vi "Script Classes in Acquire Method.vi"(8 "error in (no error)":errorcluster, 9 "Path":path, 10 "Project in":refnum<vi>, 11 "MeasurementMetaData in":refnum<class "MeasurementMetaData.lvclass">) -> (0 "error out":errorcluster, 3 "MeasurementMetaData out":refnum<class "MeasurementMetaData.lvclass">)   [LabVIEW 2016, in "MeasurementMetaData.lvclass"]
uses:
  MeasurementMetaData.lvclass
  MeasurementMetaData.lvclass/MeasurementMetaData.ctl
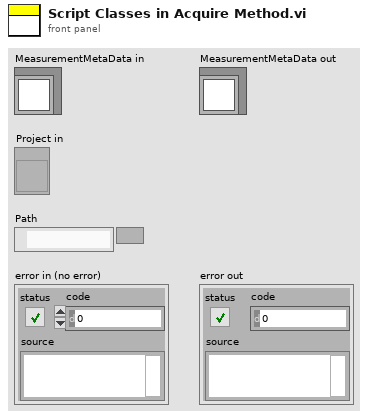
[diagram p1: front panel]
types:
  T1 = typedef "MeasurementMetaData.lvclass/Plugin Settings.ctl" = cluster{"Override Configure Method":bool, "Generate Custom Results Object":bool, "Override Measure Method":bool, "Override Close Method":bool, "Scope?":bool, "DMM?":bool, "FGEN?":bool, "PSU?":bool, "Acquisition Mode":enum16{"Continuous", "Single-Shot"}}
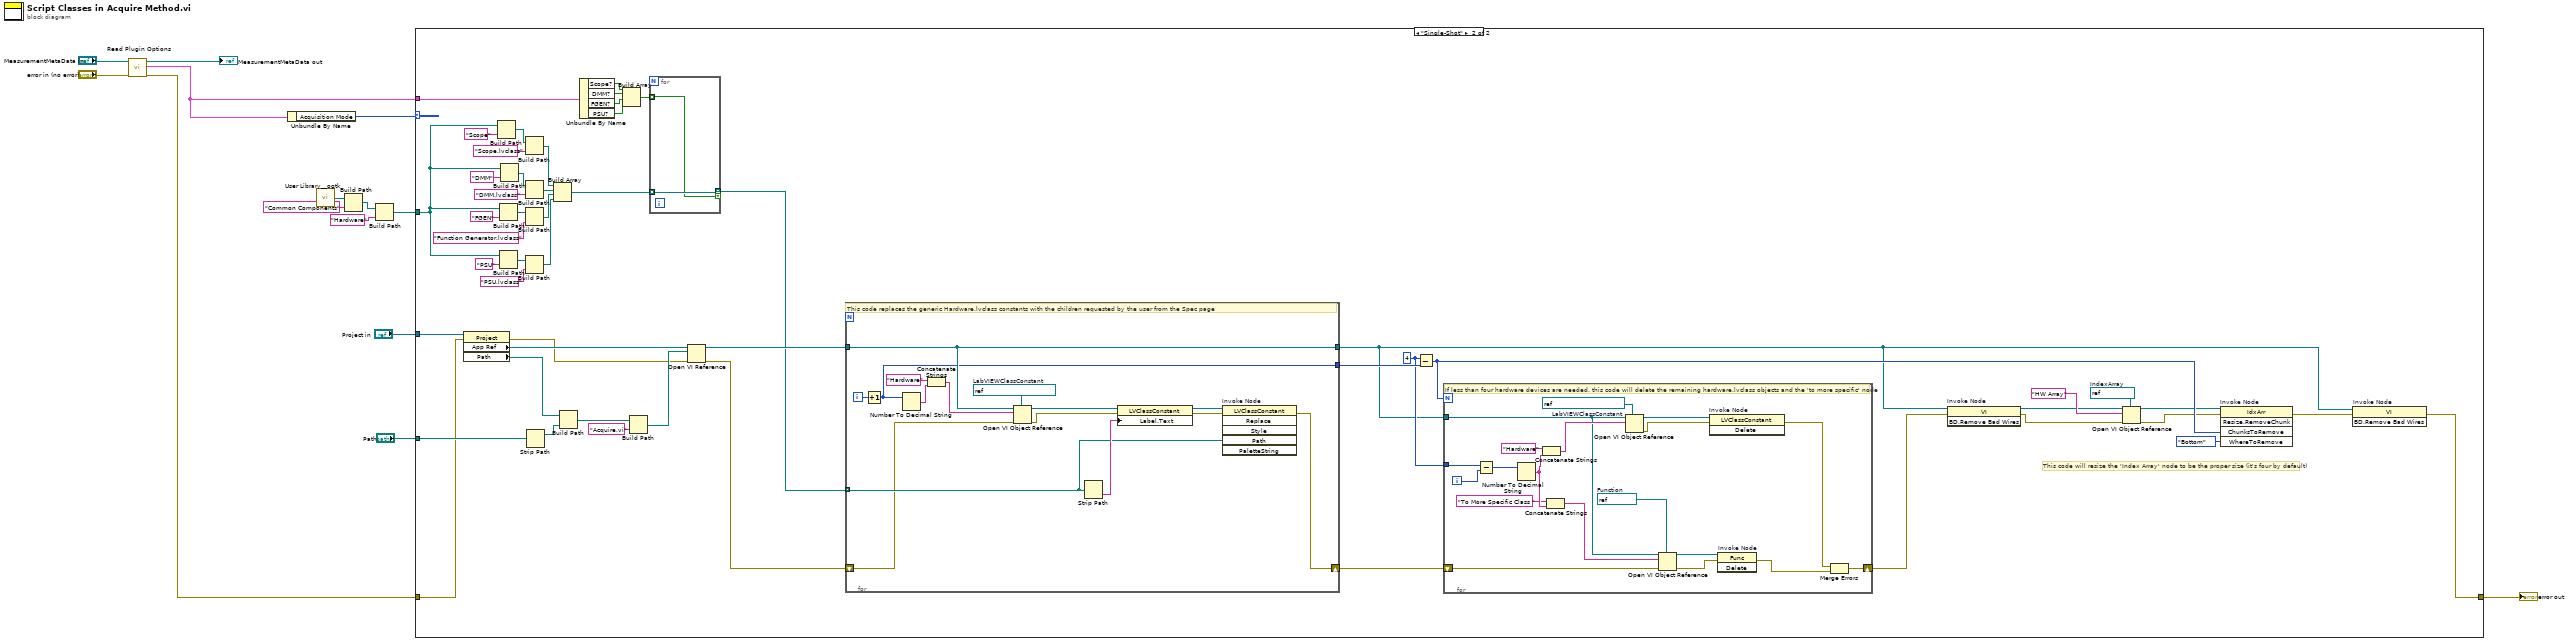
[diagram p0: block diagram]
diagram:
  n1 = call "Read Plugin Options.vi"("error in (no error)"="error in (no error)", "MeasurementMetaData in"="MeasurementMetaData in") -> ("error out"=w1:errorcluster, "Plugin Options"=w8:T1, "MeasurementMetaData out"=→"MeasurementMetaData out":refnum<class "MeasurementMetaData.lvclass">)  [unwired: 7 in]
  n2 = Unbundle By Name(w8) -> ("Acquisition Mode"=w9:enum16{"Continuous", "Single-Shot"})
  n3 = call <userlib>:"User Library__ogtk.vi"() -> ("User Library (+ Relative)"=w13:path)  [unwired: 1 in]
  n4 = Build Path(base path=w13, name or relative path="Common Components") -> (appended path=w11:path)
  n5 = Build Path(base path=w11, name or relative path="Hardware") -> (appended path=w14:path)
  n6 = case shown="\"Single-Shot\"" w9 {
    tunnel: "Project in" -> [_ w67]
    tunnel: "Path" -> [_ w64]
    tunnel: w8 -> [_ w52]
    tunnel: w14 -> [_ w39]
    tunnel: [w15 w25] -> w2
    tunnel: w1 -> [w15 w24]
    frame "Continuous" {
    }
    frame "Single-Shot" {
      w32 = refnum<vi> refnum  # IndexArray
      w29 = 4 ("x")
      # "This code will resize the 'Index Array' node to be the proper size (it's four by default)"
      n7 = property class="Project"(reference=w67, error in=w24) -> (error out=w22:errorcluster, "App Ref"=w61:refnum<vi>, "Path"=w65:path)  [unwired: 1 out]
      n8 = Build Path(base path=w39, name or relative path="Scope") -> (appended path=w48:path)
      n9 = Build Path(base path=w39, name or relative path="FGEN") -> (appended path=w50:path)
      n10 = Build Path(base path=w39, name or relative path="PSU") -> (appended path=w51:path)
      n11 = Build Path(base path=w39, name or relative path="DMM") -> (appended path=w49:path)
      n12 = Build Path(base path=w48, name or relative path="Scope.lvclass") -> (appended path=w47:path)
      n13 = Build Path(base path=w49, name or relative path="DMM.lvclass") -> (appended path=w46:path)
      n14 = Build Path(base path=w50, name or relative path="Function Generator.lvclass") -> (appended path=w45:path)
      n15 = Build Path(base path=w51, name or relative path="PSU.lvclass") -> (appended path=w44:path)
      n16 = Strip Path(path=w64) -> (stripped path=w66:path)  [unwired: 1 out]
      n17 = Build Array "Build Array"(w47, w46, w45, w44) -> (w57:path[])
      n18 = Build Path(base path=w65, name or relative path=w66) -> (appended path=w63:path)
      n19 = Unbundle By Name "Unbundle By Name"(w52) -> ("Scope?"=w58:bool, "DMM?"=w55:bool, "FGEN?"=w54:bool, "PSU?"=w53:bool)
      n20 = Build Array(w58, w55, w54, w53) -> (w56:bool[])
      n21 = Build Path(base path=w63, name or relative path="Acquire.vi") -> (appended path=w60:path)
      n22 = for {
        tunnel: w56 -> [w102] mode=indexing
        tunnel: w57 -> [w103] mode=indexing
        tunnel: [w103] -> w34 mode=indexing if=w102
      }
      n23 = Open VI Reference(application reference (local)=w61, vi path=w60, error in (no error)=w22) -> (vi reference=w59:refnum<vi>, error out=w21:errorcluster)  [unwired: 3 in]
      n24 = for {
        tunnel: w59 -> [w94]
        tunnel: w34 -> [w99] mode=indexing
        tunnel: [w93] -> w33
        tunnel: [w94] -> w19
        shift-right: [w88] -> w23
        shift-left: w21 -> [w87]
        i -> [w95]
        w101 = refnum<vi> refnum  # LabVIEWClassConstant
        # "This code replaces the generic Hardware.lvclass constants with the children requested by the user from the Spec page"
        n25 = Increment(x=w95) -> (x+1=w93:i32)
        n26 = Number To Decimal String(number=w93) -> (decimal integer string=w97:string)  [unwired: 1 in]
        n27 = Concatenate Strings("Hardware" ("name/order"), w97) -> (w96:string)
        n28 = Open VI Object Reference(7:w101, 8:w87, 10:w96, 11:w94) -> (0:w90:errorcluster, 3:w92:refnum<vi>)
        n29 = Strip Path(path=w99) -> (name=w100:string)  [unwired: 1 out]
        n30 = property class="LVClassConstant"(reference=w92, error in=w90, "Label.Text"=w100) -> (reference out=w91:refnum<vi>, error out=w89:errorcluster)
        n31 = invoke on="Invoke Node" class="LVClassConstant" method="Replace"(reference=w91, error in=w89, "Path"=w99) -> (error out=w88:errorcluster)  [unwired: 3 in, 5 out]
      }
      n32 = Subtract(x=w29, y=w33) -> (x-y=w28:i32)
      n33 = for {
        N: w28 -> [_]
        tunnel: w29 -> [w86]
        tunnel: w19 -> [w76]
        shift-right: [w69] -> w17
        shift-left: w23 -> [w68]
        i -> [w85]
        w75 = refnum<vi> refnum  # Function
        w81 = refnum<vi> refnum  # LabVIEWClassConstant
        # "If less than four hardware devices are needed, this code will delete the remaining hardware.lvclass objects and the 'to more specific' node"
        n34 = Subtract(x=w86, y=w85) -> (x-y=w82:i32)
        n35 = Number To Decimal String(number=w82) -> (decimal integer string=w79:string)  [unwired: 1 in]
        n36 = Concatenate Strings("Hardware" ("name/order"), w79) -> (w84:string)
        n37 = Concatenate Strings("To More Specific Class " ("string"), w79) -> (w77:string)
        n38 = Open VI Object Reference(7:w81, 10:w84, 11:w76) -> (0:w73:errorcluster, 3:w80:refnum<vi>)  [unwired: 1 in]
        n39 = Open VI Object Reference(7:w75, 8:w68, 10:w77, 11:w76) -> (0:w72:errorcluster, 3:w74:refnum<vi>)
        n40 = invoke on="Invoke Node" class="LVClassConstant" method="Delete"(reference=w80, error in=w73) -> (error out=w71:errorcluster)  [unwired: 1 in, 2 out]
        n41 = invoke on="Invoke Node" class="Func" method="Delete"(reference=w74, error in=w72) -> (error out=w70:errorcluster)  [unwired: 1 in, 2 out]
        n42 = Merge Errors(w71, w70) -> (w69:errorcluster)
      }
      n43 = invoke on="Invoke Node" class="VI" method="BD.Remove Bad Wires"(reference=w19, error in=w17) -> (reference out=w18:refnum<vi>, error out=w16:errorcluster)  [unwired: 1 in, 1 out]
      n44 = Open VI Object Reference(7:w32, 8:w16, 10:"HW Array" ("name/order"), 11:w18) -> (0:w27:errorcluster, 3:w20:refnum<vi>)
      n45 = invoke on="Invoke Node" class="IdxArr" method="Resize.RemoveChunk"(reference=w20, error in=w27, "ChunksToRemove"=w28, "WhereToRemove"=enum8{"Bottom", "Top"}."Bottom" ("Where To Remove")) -> (error out=w26:errorcluster)  [unwired: 1 in, 4 out]
      n46 = invoke on="Invoke Node" class="VI" method="BD.Remove Bad Wires"(reference=w19, error in=w26) -> (error out=w25:errorcluster)  [unwired: 1 in, 2 out]
    }
  }
  "error out" <- w2
